vi "Drawing Pad.vi"(8 "entrée d'erreur":errorcluster) -> (0 "sortie d'erreur":errorcluster, 3 "Données image":cluster{"Rouge":u8, "Vert":u8, "Bleu":u8}[][](array[cluster]))   [LabVIEW 2009]
uses:
  <vilib>/Utility/cursorutil.llb/Set Cursor (Icon Pict).vi
panel:
  in  "Effacer":bool
  in  "Couleur du crayon":u32(colorbox)
  in  "Terminer":bool
  out "Image":picture
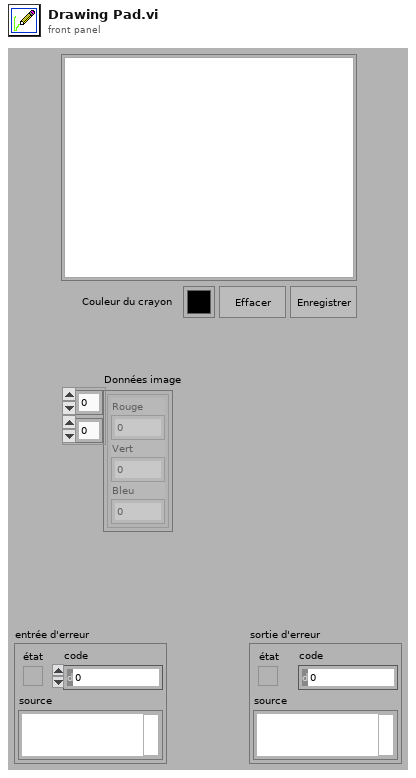
[diagram p1: front panel]
types:
  T1 = typedef "LVPoint32TypeDef.ctl" = cluster{"Horizontal":i32, "Vertical":i32}
  T2 = typedef "LVBoundsTypeDef.ctl" = cluster{"Width":u32, "Height":u32}
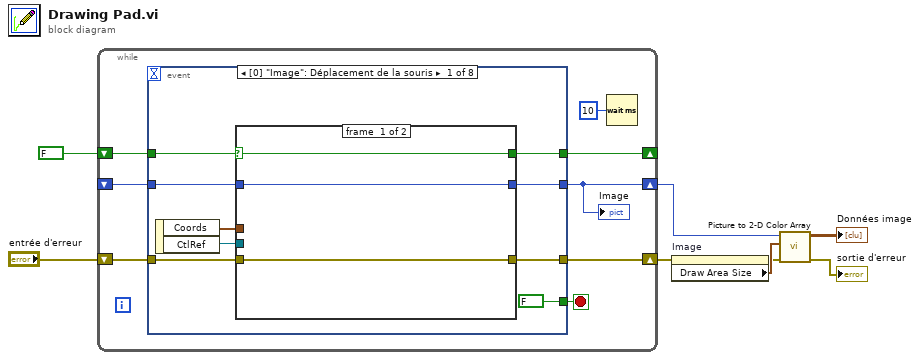
[diagram p0: block diagram]
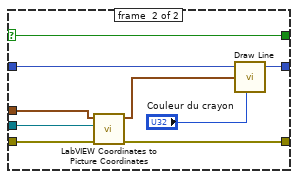
[diagram p2: hidden frame]
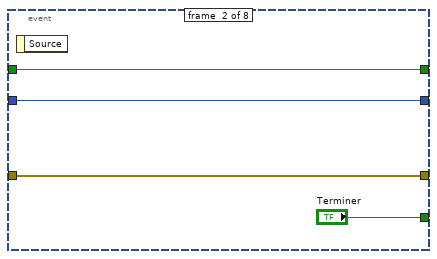
[diagram p3: hidden frame]
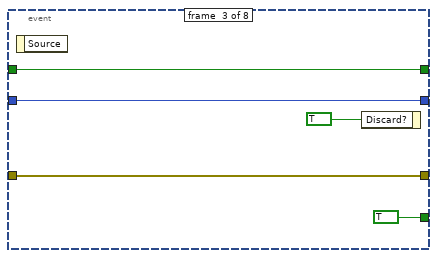
[diagram p4: hidden frame]
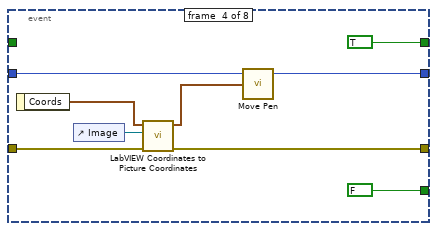
[diagram p5: hidden frame]
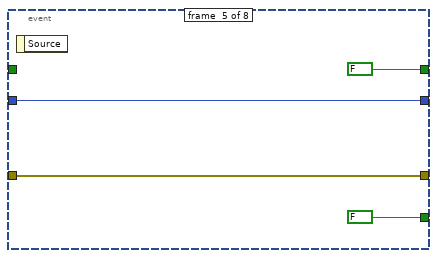
[diagram p6: hidden frame]
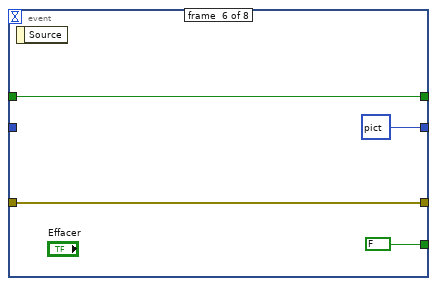
[diagram p7: hidden frame]
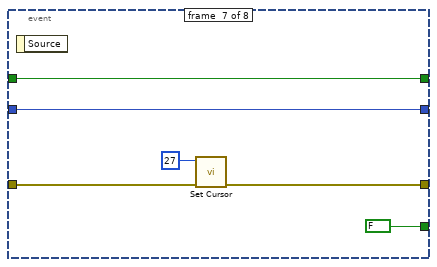
[diagram p8: hidden frame]
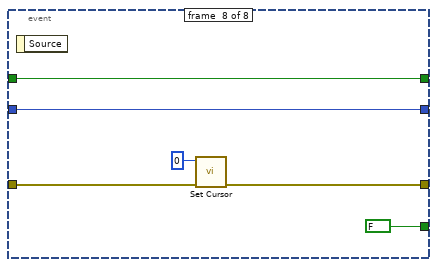
[diagram p9: hidden frame]
diagram:
  n1 = while "Boucle While" {
    shift-right: [w14] -> _
    shift-left: FALSE -> [w16]
    shift-right: [w13] -> w2
    shift-left: "entrée d'erreur" -> [w12]
    shift-right: [w10] -> w5
    shift-left: _ -> [w11]
    stop <- w15 stop-if-true
    n2 = event "Structure Événement" shown="[0] \"Image\": Déplacement de la souris" {
      selector: _ -> [_ _ _ _ _ _ _ _]
      dyn-events: _ -> [_ _ _ _ _ _ _ _]
      timeout: _ -> [_ _ _ _ _ _ _ _]
      tunnel: w16 -> [w25 w40 w46 _ _ w62 w65 w72]
      tunnel: [FALSE ("Done") "Terminer" TRUE ("Done") FALSE FALSE FALSE ("Done") FALSE ("Done") FALSE ("Done")] -> w15
      tunnel: [w24 w40 w46 TRUE FALSE w62 w65 w72] -> w14
      tunnel: [w18 w38 w44 w48 w56 w61 w68 w74] -> w13
      tunnel: w12 -> [w19 w38 w44 w49 w56 w61 w67 w73]
      tunnel: [w23 w39 w45 w50 w57 picture data[5B] ("new picture") w66 w71] -> w10
      tunnel: w11 -> [w22 w39 w45 w51 w57 _ w66 w71]
      event #0 {
        n3 = event-data() -> ("Coords"=w21:T1, "CtlRef"=w20:refnum<vi>)  [unwired: 1 out]
        n4 = case shown="Vrai" w25 {
          selector: w25 -> [w28 w37]
          tunnel: [w28 w37] -> w24
          tunnel: [w27 w36] -> w23
          tunnel: w22 -> [w27 w35]
          tunnel: w21 -> [_ w30]
          tunnel: w20 -> [_ w31]
          tunnel: w19 -> [w26 w33]
          tunnel: [w26 w32] -> w18
          frame #0 {
          }
          frame #1 {
            n5 = call "LabVIEW Coordinates to Picture Coordinates.vi"("entrée d'erreur"=w33, "RéfCmde"=w31, "Coordonnées LabVIEW"=w30) -> ("sortie d'erreur"=w32:errorcluster, "Coordonnées de la commande image"=w29:cluster{"Horizontale":i32, "Verticale":i32})  [unwired: 3 in, 4 out]
            n6 = call <vilib>:"Draw Line.vi"("picture"=w35, "end point"=w29, "color(black)"="Couleur du crayon") -> ("new picture"=w36:picture)  [unwired: 2 in, 4 out]
          }
        }
      }
      event #1 {
        n7 = event-data() -> ()  [unwired: 2 out]
      }
      event #2 {
        n8 = event-data() -> ()  [unwired: 2 out]
        n9 = event-data("Discard?"=TRUE) -> ()  [unwired: 1 in, 1 out]
      }
      event #3 {
        n10 = event-data() -> ("Coords"=w53:T1)  [unwired: 1 out]
        n11 = control-ref of="Image"() -> (w52:refnum<vi>)
        n12 = call "LabVIEW Coordinates to Picture Coordinates.vi"("entrée d'erreur"=w49, "RéfCmde"=w52, "Coordonnées LabVIEW"=w53) -> ("sortie d'erreur"=w48:errorcluster, "Coordonnées de la commande image"=w47:cluster{"Horizontale":i32, "Verticale":i32})  [unwired: 7 out]
        n13 = call <vilib>:"Move Pen.vi"("new position"=w47, "picture"=w51) -> ("new picture"=w50:picture)  [unwired: 1 in, 2 out]
      }
      event #4 {
        n14 = event-data() -> ()  [unwired: 2 out]
      }
      event #5 {
        n15 = event-data() -> ()  [unwired: 2 out]
      }
      event #6 {
        n16 = event-data() -> ()  [unwired: 2 out]
        n17 = call-poly <vilib>:"Set Cursor.vi"("error in (no error)"=w67, "icon"=u16 27) -> ("error out"=w68:errorcluster)  [unwired: 1 in, 8 out]
      }
      event #7 {
        n18 = event-data() -> ()  [unwired: 2 out]
        n19 = call-poly <vilib>:"Set Cursor.vi"("error in (no error)"=w73, "icon"=u16 0) -> ("error out"=w74:errorcluster)  [unwired: 1 in, 8 out]
      }
    }
    "Image" <- w10
    n20 = Wait (ms) ("Attendre (ms)")(milliseconds to wait=u32 10) -> ()  [unwired: 1 out]
  }
  n21 = property on="Image" class="Pict"(error in=w2) -> (error out=w1:errorcluster, "Draw Area Size"=w3:T2)  [unwired: 1 in, 1 out]
  n22 = call "Picture to 2-D Color Array.vi"("entrée d'erreur"=w1, "cluster d'entrée"=w3, "image"=w5) -> ("sortie d'erreur"=→"sortie d'erreur":errorcluster, "Tableau de couleurs"=→"Données image":cluster{"Rouge":u8, "Vert":u8, "Bleu":u8}[][])  [unwired: 7 out]
